vi "Initialize Increment.vi"(8 "error in (no error)":errorcluster, 11 "Numeric Data Type in":refnum<class "Numeric Data Type.lvclass">) -> (0 "error out":errorcluster, 3 "Numeric Data Type (dup)":refnum<class "Numeric Data Type.lvclass">)   [LabVIEW 2018, in "Numeric Data Type.lvclass"]
uses:
  Numeric Data Type.lvclass
  Numeric Data Type.lvclass/Numeric Data Type.ctl
  Reference Increment.vi
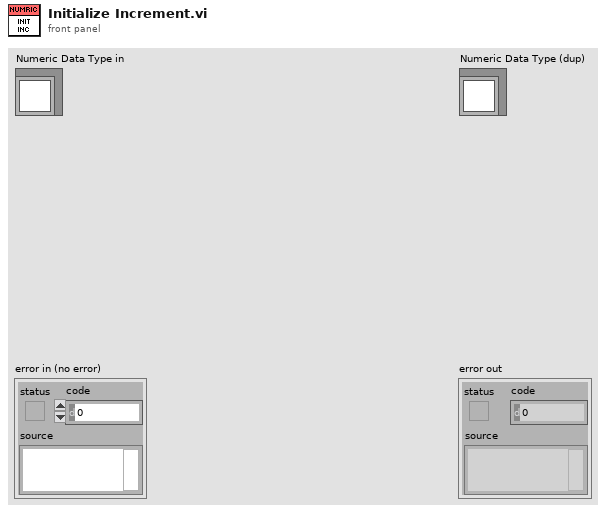
[diagram p1: front panel]
types:
  T1 = typedef "Numeric Data Type.lvclass/Representation Enum.ctl" = enum16{"Extended (EXT)", "Double (DBL)", "Single (SGL)", "Fixed-Point (FXP)", "Quad Integer (I64)", "Long Integer (I32)", "Word Integer (I16)", "Byte Integer (I8)", "Unsigned Quad (U64)", "Unsigned Long (U32)", "Unsigned Word (U16)", "Unsigned Byte (U8)", "Complex Extended (CXT)", "Complex Double (CDB)", "Complex Single (CSG)"}
  T2 = enum8{"Enabled", "Disabled", "Disabled and Grayed Out"}
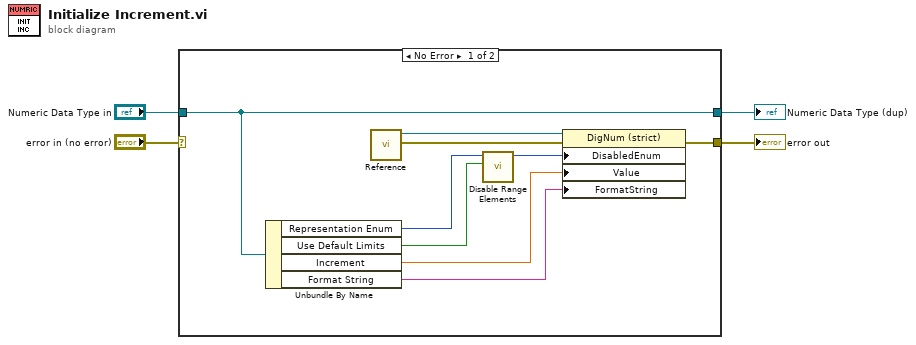
[diagram p0: block diagram]
diagram:
  n1 = case shown="No Error" "error in (no error)" {
    selector: "error in (no error)" -> [_ w15]
    tunnel: [w5 w15] -> w3
    tunnel: [w11 w14] -> w1
    tunnel: "Numeric Data Type in" -> [w11 w14]
    frame No Error {
      n2 = Unbundle By Name(w11) -> ("Representation Enum"=w8:T1, "Use Default Limits"=w7:bool, "Increment"=w9:dbl, "Format String"=w10:string)
      n3 = call-poly "Reference.vi"() -> ("error out"=w13:errorcluster, "Increment"=w12:refnum<vi>)  [unwired: 10 in]
      n4 = call "Disable Range Elements.vi"("Use Default Limits"=w7, "Representation Enum"=w8) -> ("Disabled?"=w6:T2)  [unwired: 9 in]
      n5 = property class="DigNum (strict)"(reference=w12, error in=w13, "DisabledEnum"=w6, "Value"=w9, "FormatString"=w10) -> (error out=w5:errorcluster)  [unwired: 1 out]
    }
    frame Error {
    }
  }
  "error out" <- w3
  "Numeric Data Type (dup)" <- w1
